vi "PH_Sixpack.Close.vi"(0 "i ref in":refnum<vi>, 5 "error in (no error)":errorcluster) -> (14 "i ref out":refnum<vi>, 19 "error out":errorcluster)   [LabVIEW 2014, in "PH_Sixpack.lvlib"]
doc: "This VI closes the I/O interface with the instrument."
uses:
  PH_Sixpack.lvlib
  instr.lib/Sixpack/Sixpack - Driver.lvlib
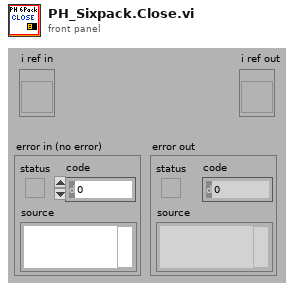
[diagram p1: front panel]
types:
  T1 = typedef "PH_Sixpack.lvlib/PH_Sixpack.i attribute.ctl" = cluster{"Information":cluster{"SixPack ID(0)":u16, "BaudRate(19200)":u16, "COM Port":enum32{"COM1", "COM2", "COM3", "COM4", "COM5", "COM6", "COM7", "COM8", "COM9"}, "HANDLE":i32}, "Serial Number":dbl, "Firmwareversion":dbl, "Axes":T2[], "Status":T14, "Axis to do a RefSearch":i32, "GUI Refs":cluster{"Information":refnum<vi>, "Serial Number":refnum<vi>, "Firmwareversion":refnum<vi>, "Status":refnum<vi>, "Axis to do a RefSearch":refnum<vi>, "Axes Configuration (Sixpack)":refnum<vi>, "Inputs":refnum<vi>, "PeriodicInterval [ms]":refnum<vi>}, "Constructor finished":bool, "Ignore Error":bool}
  T2 = typedef "PH_Sixpack.lvlib/PH_Sixpack.Axis Cluster.ctl" = cluster{"Config":T3, "To set?":cluster{"VmaxAmax":bool, "I max":bool, "VStartVminDivi":bool, "Ref Search Parameter":bool, "Stopswitch Limits":bool, "Axis Parameter":bool, "I Control":bool}}
  T3 = typedef "PH_Sixpack.lvlib/PH_Sixpack.Axis Configuration.ctl" = cluster{"VmaxAmax":T4, "I max (50%)":T5, "VStartVminDivi":T6, "Ref Search Parameter":T7, "Stopswitch Limits":T8, "Axis Parameter":T9, "I Control":T12}
  T4 = typedef "Sixpack - Driver.lvlib/VmaxAmax.ctl" = cluster{"VMax(511)":u16, "AMax(128)":u16}
  T5 = typedef "Sixpack - Driver.lvlib/PeakCurrent.ctl" = dbl
  T6 = typedef "Sixpack - Driver.lvlib/VStartVmin.ctl" = cluster{"VStart(5)":u16, "Vmin(4)":u16, "Div i (2)":enum8{"0", "1", "2", "3"}}
  T7 = typedef "Sixpack - Driver.lvlib/Ref Search Parameter.ctl" = cluster{"VRefMax(100)":u16, "DebouncingTime (22ms)":u8}
  T8 = typedef "Sixpack - Driver.lvlib/Stopswitch Limits.ctl" = cluster{"MinLeft(0)":u16, "MaxRight(1023)":u16}
  T9 = typedef "Sixpack - Driver.lvlib/Motor Parameter.ctl" = cluster{"Poslimit (6400)":u32, "P5 Bits":T10, "P6 Bits":T11}
  T10 = typedef "Sixpack - Driver.lvlib/MotorParameter_P5.ctl" = cluster{"MT_PI":bool, "MT_ROTARY":bool, "MT_AUTONULLCMD":bool, "MT_TESTNULL":bool, "MT_NULLLEFT":bool, "MT_NULLCENTRE":bool, "MT_STOPNULL":bool, "MT_FILTERSWITCH":bool}
  T11 = typedef "Sixpack - Driver.lvlib/MotorParameter_P6.ctl" = cluster{"MT_OPTIMIZEWAY":bool, "MT_FASTREF":bool, "MT_MECHREF":bool, "MT_DELAYTESTNULL":bool, "MT_STOPSOFT":bool, "MT_STOPNOREF":bool, "MT_NULLPOSITIVE":bool, "MUT_STOPFULSTEPS":bool}
  T12 = typedef "Sixpack - Driver.lvlib/Current Control.ctl" = cluster{"PowerDownDelay (500)":u16, "PowerDown (0%)":T13, "Standing (50%)":T13, "Running (75%)":T13, "Accelerating (100%)":T13}
  T13 = typedef "Sixpack - Driver.lvlib/Current.ctl" = enum8{"100%", "75%", "50%", "38%", "25%", "19%", "13%", "9%", "0%"}
  T14 = typedef "PH_Sixpack.lvlib/PH_Sixpack.Status.ctl" = enum32{"None", "Init", "Configure", "configured", "Close", "closed"}
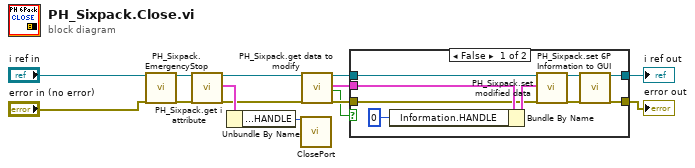
[diagram p0: block diagram]
diagram:
  n1 = call "PH_Sixpack.EmergencyStop.vi"("i ref in"="i ref in", "error in"="error in (no error)") -> ("i ref out"=w2:refnum<vi>, "error out"=w3:errorcluster)  [unwired: 15 in, 1 out]
  n2 = call "PH_Sixpack.get i attribute.vi"("i ref in"=w2, "error in (no error)"=w3) -> ("i ref out"=w8:refnum<vi>, "i attribute"=w14:T1, "error out"=w6:errorcluster)  [unwired: 15 in]
  n3 = Unbundle By Name(w14) -> ("Information.HANDLE"=w13:i32)
  n4 = call "ClosePort.vi"("handle"=w13) -> ()  [unwired: 19 in]
  n5 = call "PH_Sixpack.get data to modify.vi"("i ref in"=w8, "error in (no error)"=w6) -> ("i ref out"=w12:refnum<vi>, "i attribute"=w10:T1, "timed out"=w9:bool, "error out"=w11:errorcluster)  [unwired: 14 in]
  n6 = case shown="False" w9 {
    tunnel: [w16 w24] -> w5
    tunnel: [w17 w25] -> w7
    tunnel: w12 -> [w22 w25]
    tunnel: w11 -> [w19 w24]
    tunnel: w10 -> [w20 _]
    frame False {
      n7 = Bundle By Name(cluster=w20, "Information.HANDLE"=0) -> (w21:T1)
      n8 = call "PH_Sixpack.set modified data.vi"("i ref in"=w22, "i attribute"=w21, "error in (no error)"=w19) -> ("i ref out"=w18:refnum<vi>, "error out"=w23:errorcluster)  [unwired: 15 in]
      n9 = call "PH_Sixpack.set 6P Information to GUI.vi"("VI in"=w18, "error in (no error)"=w23) -> ("VI out"=w17:refnum<vi>, "error out"=w16:errorcluster)  [unwired: 16 in]
    }
    frame True {
      (unwired) errorcluster {"status"=FALSE, "code"=0, "source"=""} ("error out")
    }
  }
  "error out" <- w5
  "i ref out" <- w7
